vi "ex4_multi.vi"() -> ()   [LabVIEW 2022 SP3]
uses:
  C:/Program Files (x86)/National Instruments/LabVIEW 2022/examples/Connectivity/Python/support/PythonVersionsEnum.ctl
  pylabview/pythonq.lvlib
  <vilib>/Analysis/NI_AALBase.lvlib
panel:
  out "Hz Meter":dbl(knob) scale=0.0..1000.0
  out "data in buffer":i32(graph)
  out "hz_wv":dbl(graph)
  out "hz":dbl
  out "cur ref 2":string
  out "error out 2":errorcluster
  out "Wv 2":dbl(graph)
  out "cur ref":string
  out "count 1":i32
  in  "wait":u32=500
  out "Wv":dbl(graph)
  in  "stop":bool
  out "count 2":i32
  out "error out":errorcluster
  # "This example shows 2 connections to the python data ques, 1 to produce data, and one to consumer it, all in parrallel\n\nCreated by Jeff Morgan\nhttps://awakeniot.com/"
  # "https://github.com/jmor2000/labview_python_bridge"
  # "DATA IN"
  # "DATA OUT"
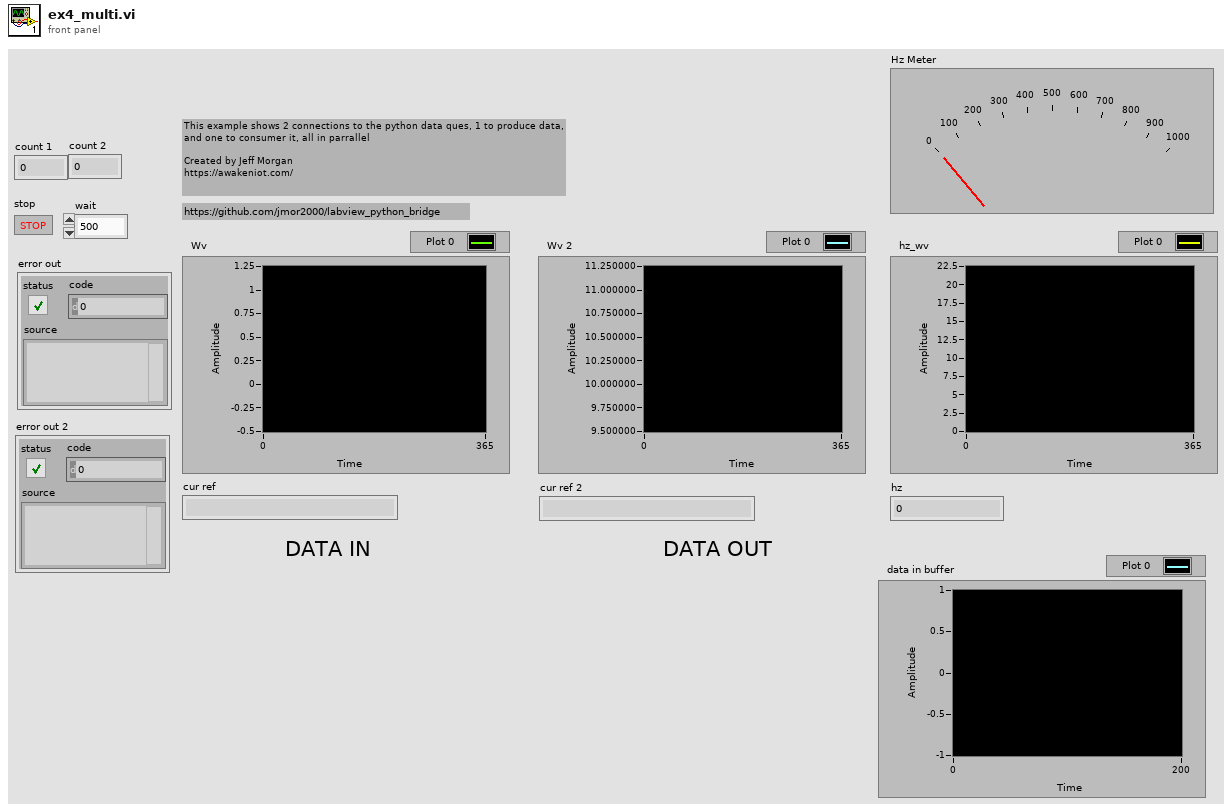
[diagram p1: front panel]
types:
  T1 = typedef "PythonVersionsEnum.ctl" = enum16{"3.6", "3.7", "3.8", "3.9"}
  T2 = typedef "pythonq.lvlib/py_cluster.ctl" = cluster{"path":path, "py":T3}
  T3 = typedef "pythonq.lvlib/py_session.ctl" = cluster{"session":refnum<k35>, "object":refnum<k38>}
  T4 = typedef "pythonq.lvlib/py_result.ctl" = cluster{"value":string, "ok":bool, "error_msg":string}
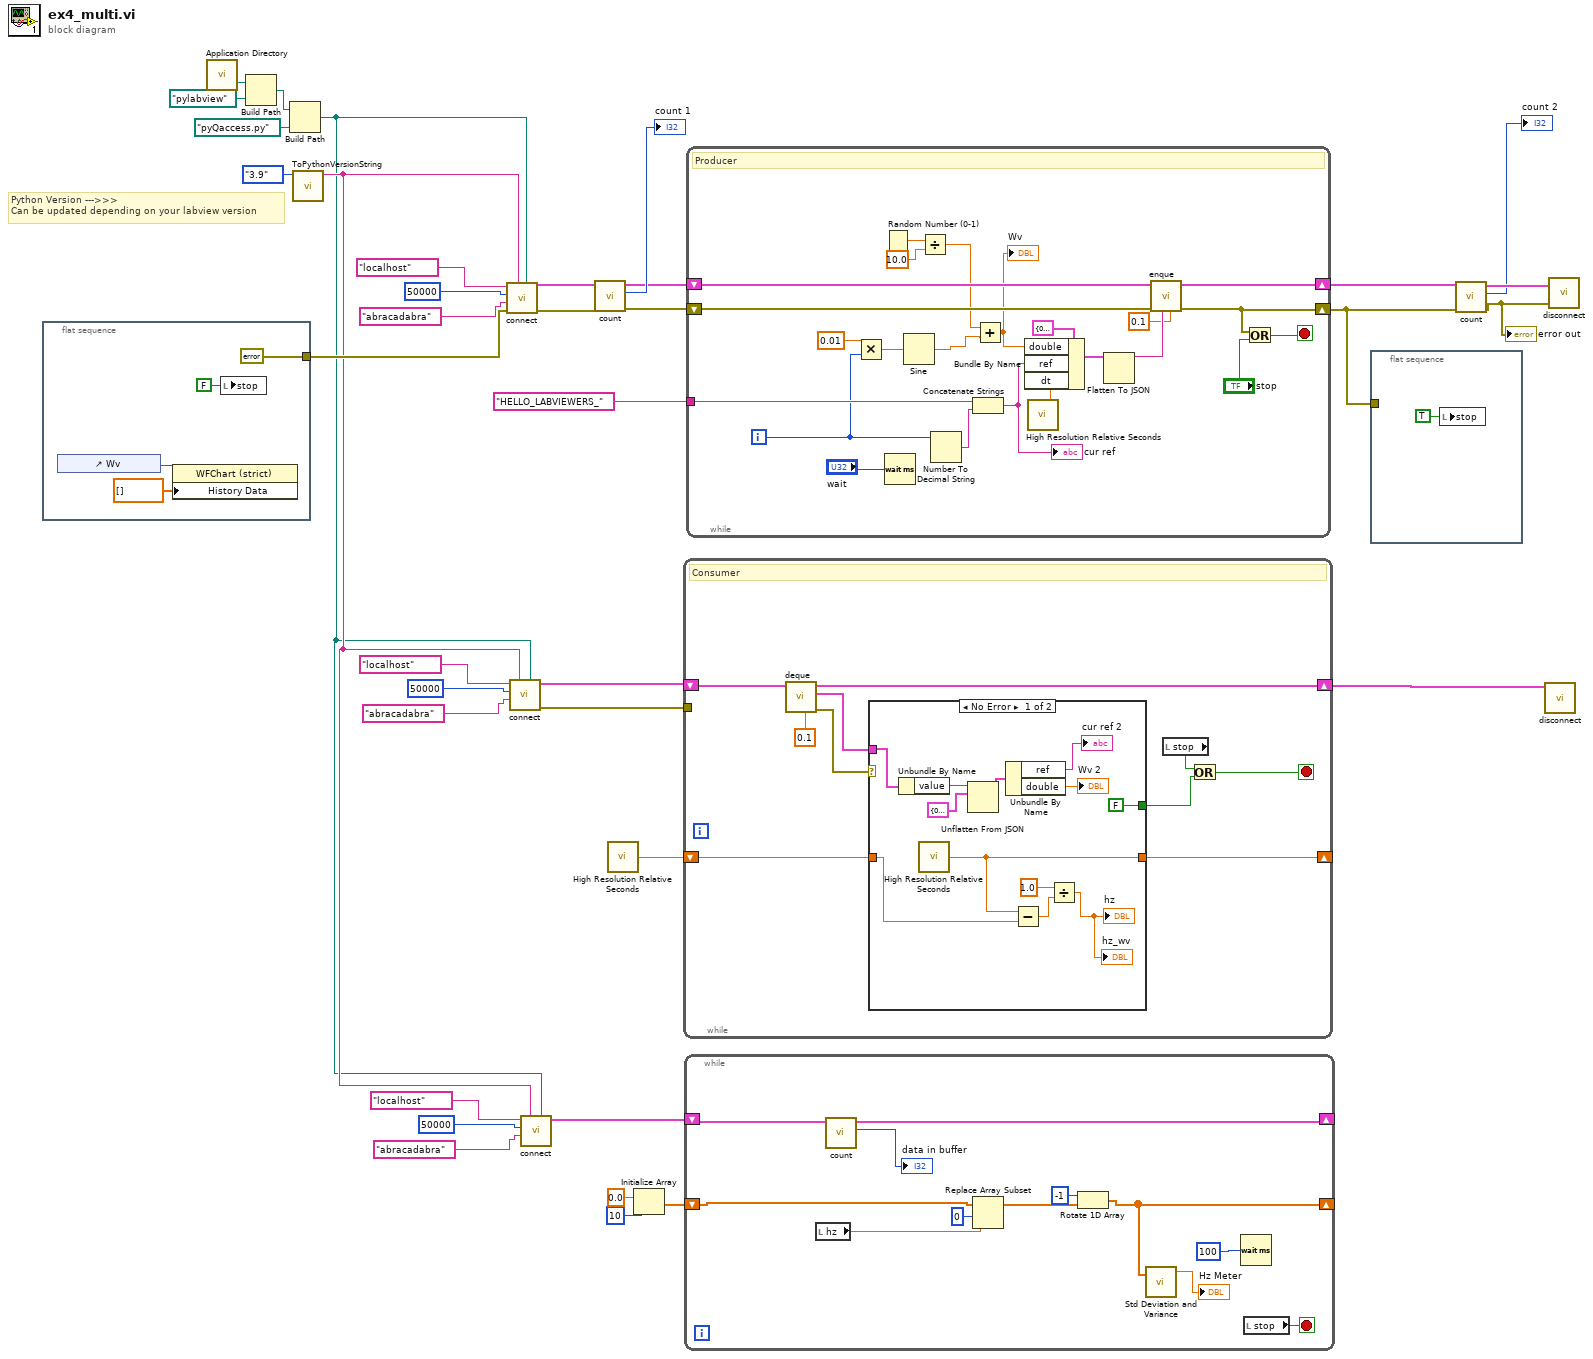
[diagram p0: block diagram]
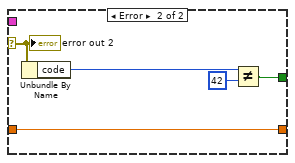
[diagram p2: hidden frame]
diagram:
  # "Python Version --->>>\nCan be updated depending on your labview version"
  n1 = flat-sequence {
    tunnel: [errorcluster {"status"=FALSE, "code"=0, "source"=""} ("error in (no error)")] -> w24
    frame #0 {
      n2 = control-ref of="Wv"() -> (w38:refnum<vi>)
      n3 = property class="WFChart (strict)"(reference=w38, "History Data"=dbl[] []) -> ()  [unwired: 1 in, 2 out]
      n4 = local write "stop"(FALSE ("stop")) -> ()
    }
  }
  n5 = call <vilib>:"Application Directory.vi"() -> ("Application Directory"=w31:path)
  n6 = Build Path(base path=w31, name or relative path=path "pylabview") -> (appended path=w32:path)
  n7 = Build Path(base path=w32, name or relative path=path "pyQaccess.py") -> (appended path=w6:path)
  n8 = call "ToPythonVersionString.vi"("python version"=PythonVersionsEnum."3.9") -> ("python version string"=w7:string)  [unwired: 10 in]
  n9 = call "connect.vi"("module path"=w6, "Python version"=w7, "error in (no error)"=w24, "password"="abracadabra", "port"=50000, "ip_address"="localhost") -> ("error out"=w26:errorcluster, "py out"=w25:T2)  [unwired: 4 in]
  n10 = call "connect.vi"("module path"=w6, "Python version"=w7, "password"="abracadabra", "port"=50000, "ip_address"="localhost") -> ("error out"=w14:errorcluster, "py out"=w15:T2)  [unwired: 5 in]
  n11 = call "connect.vi"("module path"=w6, "Python version"=w7, "password"="abracadabra", "port"=50000, "ip_address"="localhost") -> ("py out"=w5:T2)  [unwired: 5 in, 1 out]
  n12 = call "count.vi"("error in (no error)"=w26, "py in"=w25) -> ("error out"=w23:errorcluster, "count"=→"count 1":i32, "py out"=w19:T2)  [unwired: 7 in]
  n13 = call <vilib>:"High Resolution Relative Seconds.vi"() -> ("relative seconds"=w11:dbl)
  n14 = Initialize Array(0.0 ("element"), 10 ("dimension size")) -> (w4:dbl[])
  n15 = while {
    shift-right: [w49] -> w12
    shift-left: w15 -> [w50]
    tunnel: w14 -> [_]
    shift-right: [w42] -> _
    shift-left: w11 -> [w41]
    stop <- w46 stop-if-true
    # "Consumer"
    n16 = call "deque.vi"("timeout"=0.1, "py in"=w50) -> ("error out"=w47:errorcluster, "response"=w44:T4, "py out"=w49:T2)  [unwired: 6 in, 1 out]
    n17 = case shown="No Error" w47 {
      selector: w47 -> [_ w67]
      tunnel: [FALSE w64] -> w45
      tunnel: w44 -> [w61 _]
      tunnel: [w54 w63] -> w42
      tunnel: w41 -> [w55 w63]
      frame No Error {
        n18 = Unbundle By Name(w61) -> ("value"=w60:string)
        n19 = call <vilib>:"High Resolution Relative Seconds.vi"() -> ("relative seconds"=w54:dbl)
        n20 = Unflatten From JSON(JSON string=w60, type and defaults=cluster{"double":dbl, "ref":string, "dt":dbl} {"double"=0.0, "ref"="", "dt"=0.0} ("Cluster")) -> (value=w59:cluster{"double":dbl, "ref":string, "dt":dbl})  [unwired: 5 in, 1 out]
        n21 = Unbundle By Name(w59) -> ("ref"=→"cur ref 2":string, "double"=→"Wv 2":dbl)
        n22 = Subtract(x=w54, y=w55) -> (x-y=w52:dbl)
        n23 = Divide(x=1.0, y=w52) -> (x/y=→"hz" →"hz_wv":dbl)
      }
      frame Error {
        n24 = Unbundle By Name(w67) -> ("code"=w66:i32)
        n25 = Not Equal?(x=w66, y=42) -> (x != y?=w64:bool)
        "error out 2" <- w67
      }
    }
    n26 = local read "stop"() -> (w43:bool)
    n27 = Or(x=w43, y=w45) -> (x .or. y?=w46:bool)
  }
  n28 = while {
    shift-right: [w77] -> _
    shift-left: w5 -> [w78]
    shift-right: [w69] -> _
    shift-left: w4 -> [w72]
    stop <- w79 stop-if-true
    n29 = local read "hz"() -> (w74:dbl)
    n30 = call "count.vi"("py in"=w78) -> ("count"=→"data in buffer":i32, "py out"=w77:T2)  [unwired: 8 in, 1 out]
    n31 = Replace Array Subset(array=w72, new element=w74, index=0) -> (w71:dbl[])
    n32 = Rotate 1D Array(1:w71, 2:-1 ("n")) -> (0:w69:dbl[])
    n33 = call <vilib>:"Std Deviation and Variance.vi"("X"=w69) -> ("mean"=→"Hz Meter":dbl)  [unwired: 1 in, 2 out]
    n34 = Wait (ms)(milliseconds to wait=u32 100) -> ()  [unwired: 1 out]
    n35 = local read "stop"() -> (w79:bool)
  }
  n36 = while {
    shift-right: [w101] -> w13
    shift-left: w19 -> [w102]
    shift-right: [w98] -> w1
    shift-left: w23 -> [w100]
    tunnel: "HELLO_LABVIEWERS_" ("ref_prefix") -> [w96]
    i -> [w95]
    stop <- w99 stop-if-true
    # "Producer"
    n37 = Multiply(x=0.01, y=w95) -> (x*y=w88:dbl)
    n38 = Random Number (0-1)() -> (number: 0 to 1=w84:dbl)
    n39 = Wait (ms)(milliseconds to wait="wait") -> ()  [unwired: 1 out]
    n40 = Sine(x=w88) -> (sin(x)=w82:dbl)
    n41 = Divide(x=w84, y=10.0) -> (x/y=w81:dbl)
    n42 = Number To Decimal String(number=w95) -> (decimal integer string=w94:string)  [unwired: 1 in]
    n43 = Concatenate Strings(w96, w94) -> (w93:string)
    "cur ref" <- w93
    n44 = Add(x=w81, y=w82) -> (x+y=w80:dbl)
    "Wv" <- w80
    n45 = call <vilib>:"High Resolution Relative Seconds.vi"() -> ("relative seconds"=w86:dbl)
    n46 = Bundle By Name(cluster=cluster{"double":dbl, "ref":string, "dt":dbl} {"double"=0.0, "ref"="", "dt"=0.0} ("Cluster"), "double"=w80, "ref"=w93, "dt"=w86) -> (w92:cluster{"double":dbl, "ref":string, "dt":dbl})
    n47 = Flatten To JSON(anything=w92) -> (JSON string=w91:string)  [unwired: 2 in, 1 out]
    n48 = call "enque.vi"("timeout"=0.1, "data in"=w91, "error in (no error)"=w100, "py in"=w102) -> ("error out"=w98:errorcluster, "py out"=w101:T2)  [unwired: 4 in, 2 out]
    n49 = Or(x=w98, y="stop") -> (x .or. y?=w99:bool)
  }
  n50 = flat-sequence {
    tunnel: w1 -> [_]
    frame #0 {
      n51 = local write "stop"(TRUE ("stop")) -> ()
    }
  }
  n52 = call "count.vi"("error in (no error)"=w1, "py in"=w13) -> ("error out"=w21:errorcluster, "count"=→"count 2":i32, "py out"=w28:T2)  [unwired: 7 in]
  "error out" <- w21
  n53 = call "disconnect.vi"("py in"=w12) -> ()  [unwired: 10 in, 1 out]
  n54 = call "disconnect.vi"("error in (no error)"=w21, "py in"=w28) -> ()  [unwired: 9 in, 1 out]
